vi "DSF.Engine.Memory.Cache.Framework.Set Framework Configuration.vi"(8 "error in (no error)":errorcluster, 10 "Framework Configuration":refnum<class "DSF.Shared.Configuration.Framework.lvclass">, 11 "Framework Cache in":refnum<class "DSF.Engine.Memory.Cache.Framework.lvclass">) -> (0 "error out":errorcluster, 3 "Framework Cache out":refnum<class "DSF.Engine.Memory.Cache.Framework.lvclass">)   [LabVIEW 2016, in "DSF.Engine.lvlib" / "DSF.Engine.Memory.Cache.Framework.lvclass"]
uses:
  DSF.Engine.Memory.Cache.Framework.lvclass
  Shared/Classes/Framework/DSF.Shared.Configuration.Framework.lvclass
  DSF.Engine.Memory.Cache.Framework.lvclass/DSF.Engine.Memory.Cache.Framework.ctl
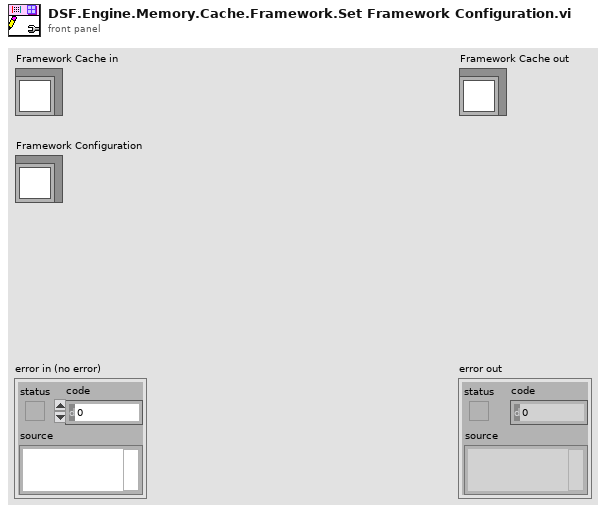
[diagram p1: front panel]
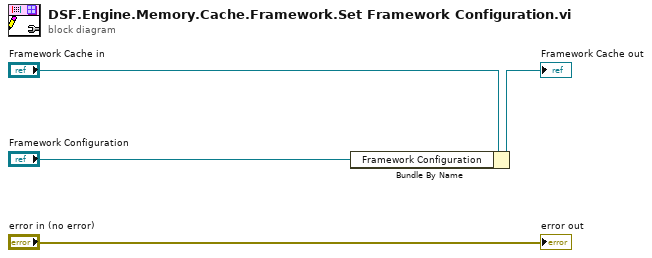
[diagram p0: block diagram]
diagram:
  n1 = Bundle By Name(cluster="Framework Cache in", "Framework Configuration"="Framework Configuration") -> (→"Framework Cache out":refnum<class "DSF.Engine.Memory.Cache.Framework.lvclass">)
  "error out" <- "error in (no error)"
